vi "Get Panel.vi"(8 "error in (no error)":errorcluster, 11 "Model Panel Logic in":refnum<class "Model Panel Logic Nested Window.lvclass">) -> (0 "error out":errorcluster, 2 "Panel":refnum<class "Panel.lvclass">, 3 "Model Panel Logic out":refnum<class "Model Panel Logic Nested Window.lvclass">)   [LabVIEW 2020, in "Form Model Configuration.lvlib" / "Model Panel Logic Nested Window.lvclass"]
uses:
  Model Panel Logic Nested Window.lvclass
  <vilib>/MGI/Panel Manager/Panel/Panel/Panel.lvclass
  Model Panel Logic Nested Window.lvclass/Model Panel Logic Nested Window.ctl
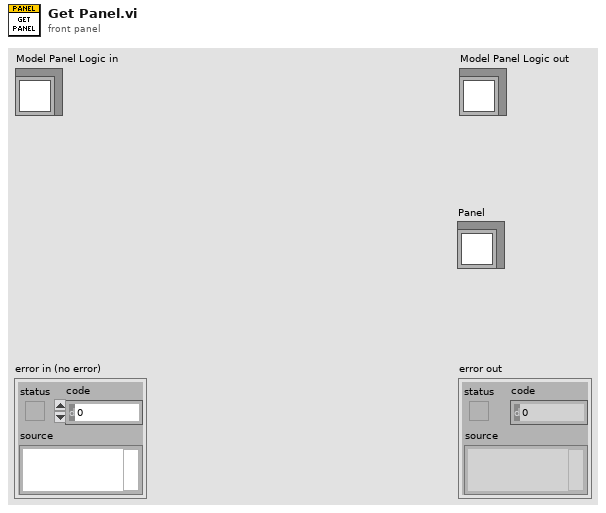
[diagram p1: front panel]
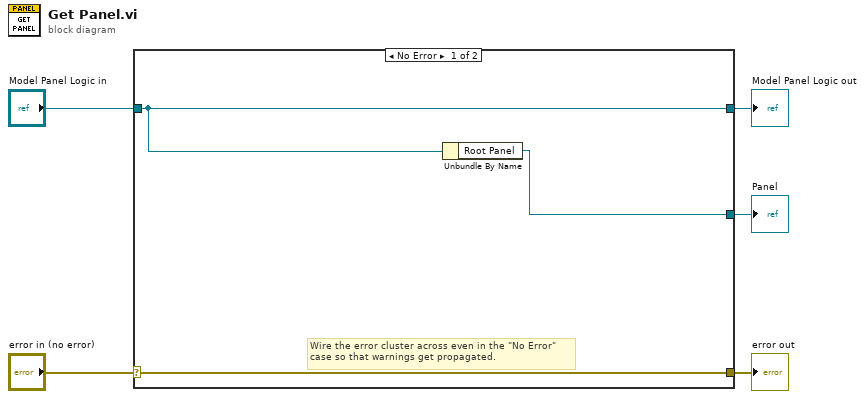
[diagram p0: block diagram]
diagram:
  n1 = case shown="No Error" "error in (no error)" {
    selector: "error in (no error)" -> [w8 w10]
    tunnel: [w8 w10] -> w4
    tunnel: [w7 w9] -> w2
    tunnel: "Model Panel Logic in" -> [w7 w9]
    tunnel: [w6 _] -> w1
    frame No Error {
      # "Wire the error cluster across even in the \"No Error\"\ncase so that warnings get propagated."
      n2 = Unbundle By Name(w7) -> ("Root Panel"=w6:refnum<class "Panel.lvclass">)
    }
    frame Error {
    }
  }
  "error out" <- w4
  "Model Panel Logic out" <- w2
  "Panel" <- w1
